vi "LIDAR Globals.vi"() -> ()   [LabVIEW 2015]
panel:
  in  "DMAQ":refnum<queue>
  in  "FileSaveQ":refnum<queue>
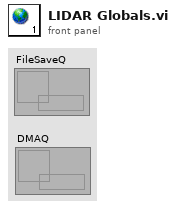
[diagram p1: front panel]
diagram:
